vi "SP Adjust Limit with Waveform Data.vi"(7 "Limit":T1={"Parameter"={"Stimulus Port"=1, "Response Port"=1}, "Format"=enum."Log Mag", "Limit Type"=enum."Upper", "Points"=[], "Referential Limit"={"Ref Limit"=FALSE, "Ref Type"=enum."Current", "Model"="", "Serial"="", "Run Type"=enum."Most Recent", "Run"=0, "Field"="", "Field Value"=""}, "Limit #"=1} {"Parameter"."Stimulus Port" min=1 step=1; "Parameter"."Response Port" min=1 step=1}, 8 "error in (no error)":errorcluster, 9 "Data Waveform":waveform(dbl)={"t0"=timestamp(0 s since 1904-01-01), "dt"=0.0, "Y"=[]}, 10 "Frequency Waveform":waveform(dbl)={"t0"=timestamp(0 s since 1904-01-01), "dt"=0.0, "Y"=[]}) -> (0 "error out":errorcluster, 5 "Modified Limit":T1={"Parameter"={"Stimulus Port"=1, "Response Port"=1}, "Format"=enum."Log Mag", "Limit Type"=enum."Upper", "Points"=[], "Referential Limit"={"Ref Limit"=FALSE, "Ref Type"=enum."Current", "Model"="", "Serial"="", "Run Type"=enum."Most Recent", "Run"=0, "Field"="", "Field Value"=""}, "Limit #"=1} {"Parameter"."Stimulus Port" min=1 step=1; "Parameter"."Response Port" min=1 step=1})   [LabVIEW 2011]
uses:
  TypeDefs/SP Limit.ctl
  TypeDefs/SP Parameter.ctl
  TypeDefs/SP Format.ctl
  TypeDefs/SP Limit Type.ctl
  TypeDefs/SP Limit Point.ctl
  Test Referential Limit.ctl
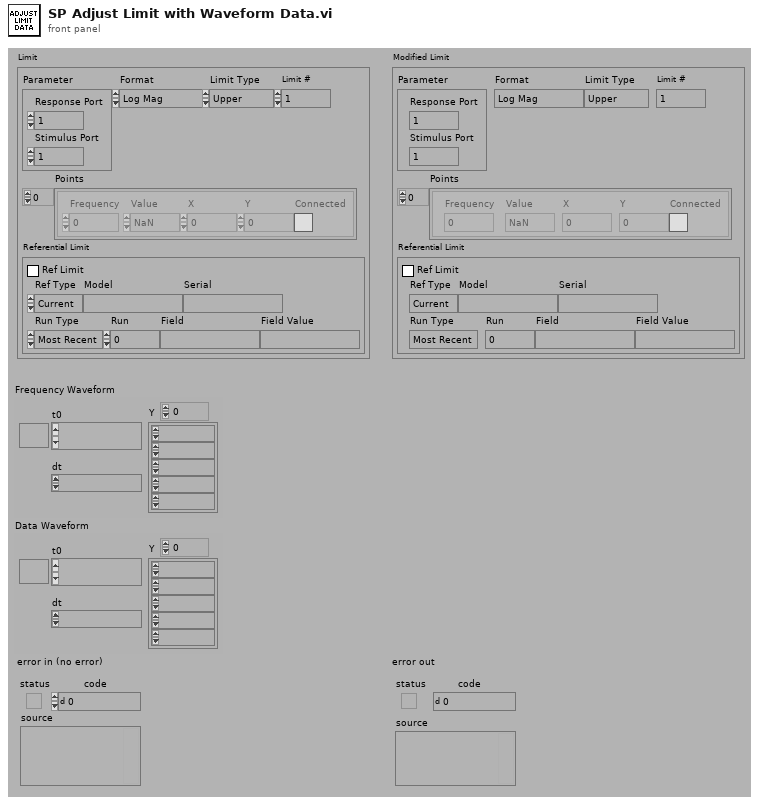
[diagram p1: front panel]
types:
  T1 = typedef "SP Limit.ctl" = cluster{"Parameter":T2, "Format":T3, "Limit Type":T4, "Points":T5[], "Referential Limit":T6, "Limit #":i8}
  T2 = typedef "SP Parameter.ctl" = cluster{"Stimulus Port":i8, "Response Port":i8}
  T3 = typedef "SP Format.ctl" = enum16{"Log Mag", "Lin Mag", "SWR", "Phase", "Expanded Phase", "Delay", "Insertion Loss", "Isolation", "Return Loss"}
  T4 = typedef "SP Limit Type.ctl" = enum16{"Upper", "Lower", "Delta", "Filter", "Referential"}
  T5 = typedef "SP Limit Point.ctl" = cluster{"Frequency":dbl, "Value":dbl, "X":dbl, "Y":dbl, "Connected":bool}
  T6 = typedef "Test Referential Limit.ctl" = cluster{"Ref Limit":bool, "Ref Type":enum16{"Current", "Specify"}, "Model":string, "Serial":string, "Run Type":enum16{"Most Recent", "Run #", "Match Field"}, "Run":i32, "Field":string, "Field Value":string}
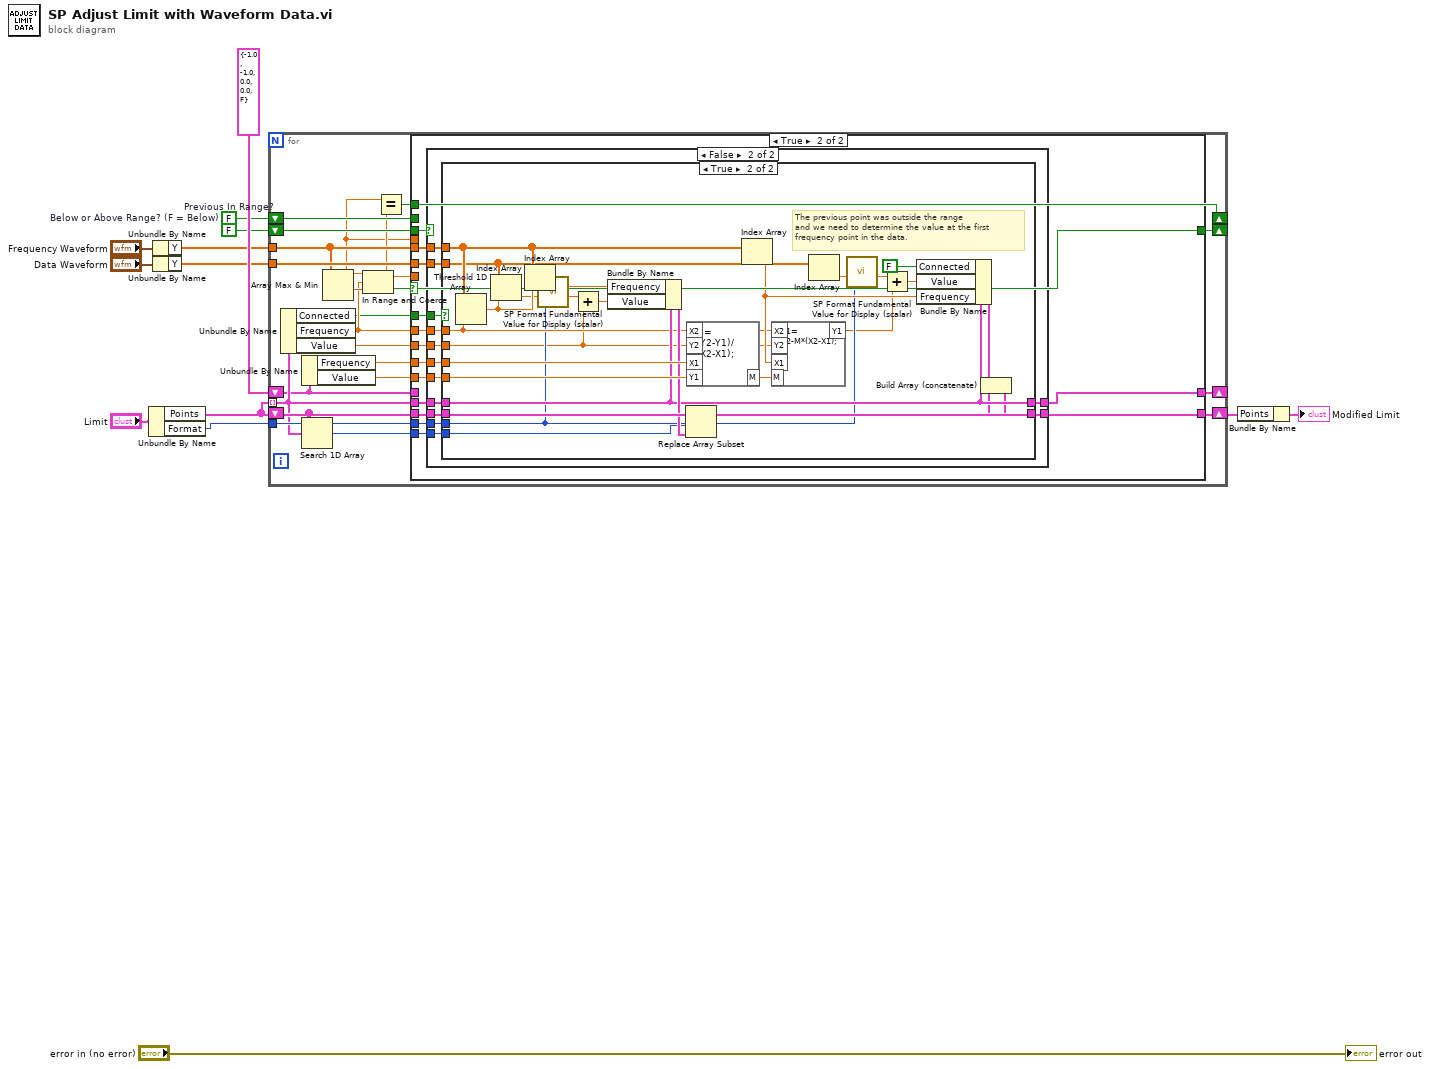
[diagram p0: block diagram]
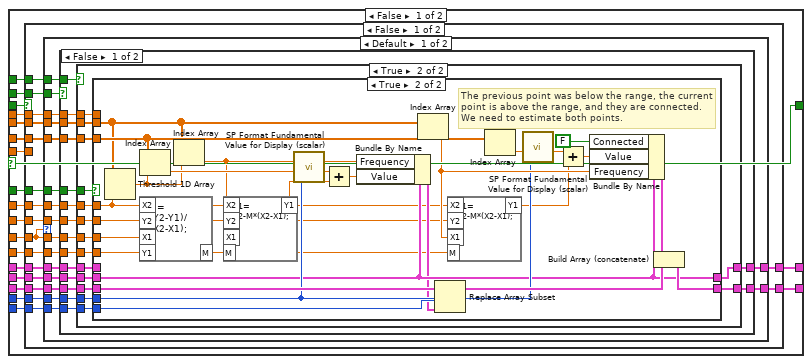
[diagram p2: hidden frame]
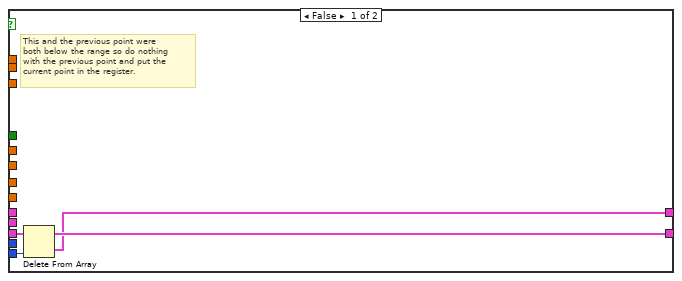
[diagram p3: hidden frame]
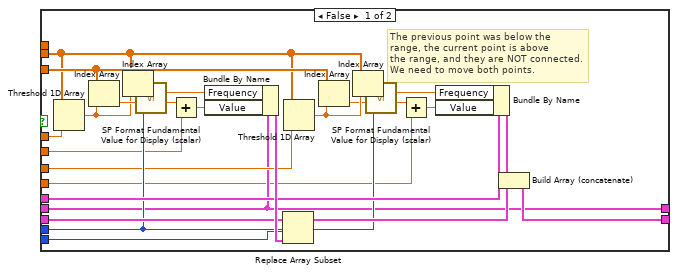
[diagram p4: hidden frame]
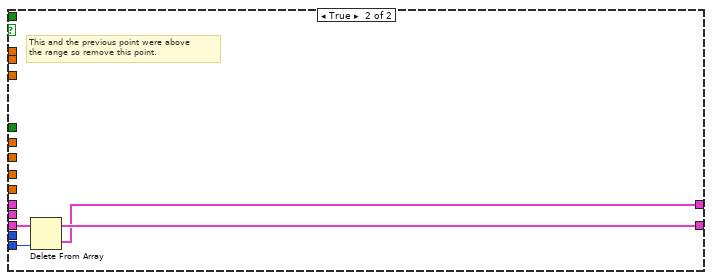
[diagram p5: hidden frame]
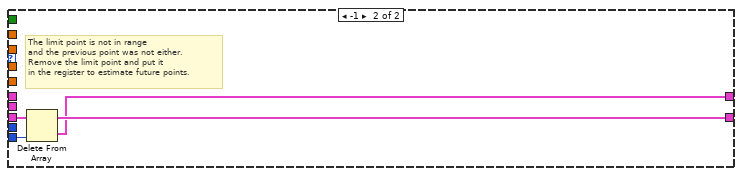
[diagram p6: hidden frame]
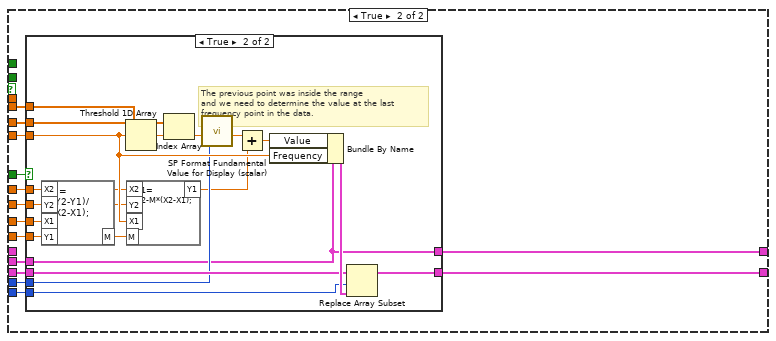
[diagram p7: hidden frame]
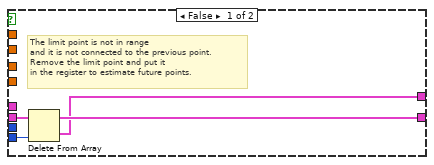
[diagram p8: hidden frame]
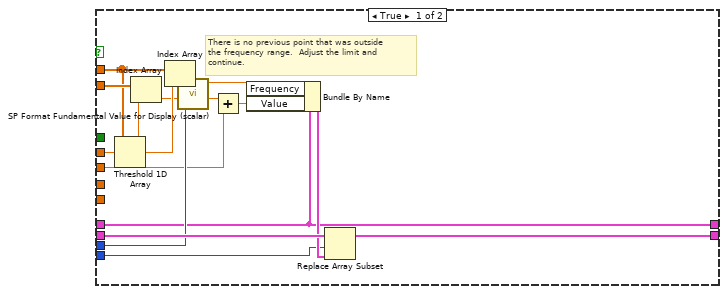
[diagram p9: hidden frame]
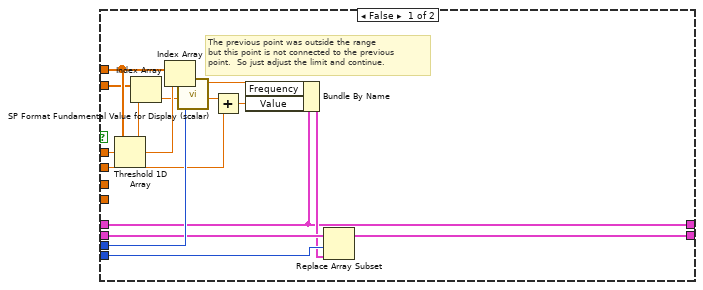
[diagram p10: hidden frame]
diagram:
  w2 = FALSE  # Below or Above Range? (F = Below)
  w3 = FALSE  # Previous In Range?
  n1 = Unbundle By Name("Limit") -> ("Points"=w7:T5[], "Format"=w6:T3)
  n2 = Unbundle By Name("Frequency Waveform") -> ("Y"=w4:dbl[])
  n3 = Unbundle By Name("Data Waveform") -> ("Y"=w1:dbl[])
  n4 = for {
    tunnel: w4 -> [w32]
    tunnel: w1 -> [w35]
    tunnel: w7 -> [w27] mode=indexing
    shift-right: [w33] -> w10
    shift-left: w7 -> [w26]
    tunnel: w6 -> [w28]
    shift-right: [w24] -> _
    shift-left: T5 {"Frequency"=-1.0, "Value"=-1.0, "X"=0.0, "Y"=0.0, "Connected"=FALSE} ("Point") -> [w14]
    shift-right: [w22] -> _
    shift-left: w3 -> [w23]
    shift-right: [w16] -> _
    shift-left: w2 -> [w18]
    n5 = Unbundle By Name(w27) -> ("Connected"=w19:bool, "Frequency"=w30:dbl, "Value"=w34:dbl)
    n6 = Unbundle By Name(w14) -> ("Frequency"=w21:dbl, "Value"=w20:dbl)
    n7 = Search 1D Array(1D array=w26, element=w27) -> (index of element=w25:i32)  [unwired: 1 out]
    n8 = Array Max & Min(array=w32) -> (max value=w15:dbl, min value=w31:dbl)  [unwired: 2 out]
    n9 = In Range and Coerce(upper limit=w15, x=w30, lower limit=w31) -> (coerced(x)=w17:dbl, In Range?=w29:bool)
    n10 = Equal?(x=w15, y=w17) -> (x = y?=w16:bool)
    n11 = case shown="True" w29 {
      selector: w29 -> [w41 w223]
      tunnel: w35 -> [w51 w236]
      tunnel: w34 -> [w54 w230]
      tunnel: w26 -> [w47 w232]
      tunnel: [w46 w231] -> w33
      tunnel: w32 -> [w50 w234]
      tunnel: w30 -> [w53 w235]
      tunnel: w27 -> [w55 w233]
      tunnel: w28 -> [w49 w229]
      tunnel: w25 -> [w48 w228]
      tunnel: [w45 w224] -> w24
      tunnel: w17 -> [w52 _]
      tunnel: w23 -> [w44 w227]
      tunnel: [w41 w223] -> w22
      tunnel: w21 -> [w42 w226]
      tunnel: w20 -> [w43 w225]
      tunnel: w19 -> [w40 w222]
      tunnel: w18 -> [w39 _]
      tunnel: w16 -> [w38 _]
      tunnel: w15 -> [w37 _]
      tunnel: w14 -> [w36 _]
      frame False {
        n12 = case shown="False" w44 {
          tunnel: w43 -> [w66 w188]
          tunnel: w55 -> [w58 w198]
          tunnel: w54 -> [w68 w197]
          tunnel: w53 -> [w67 w196]
          tunnel: w52 -> [_ w195]
          tunnel: w51 -> [w60 w194]
          tunnel: w50 -> [w59 w193]
          tunnel: w49 -> [w63 w192]
          tunnel: w48 -> [w69 w191]
          tunnel: w47 -> [w72 w190]
          tunnel: w42 -> [w65 w189]
          tunnel: [w71 w187] -> w46
          tunnel: [w70 w186] -> w45
          tunnel: w40 -> [w61 w185]
          tunnel: w39 -> [w64 _]
          tunnel: w38 -> [w62 _]
          tunnel: w37 -> [w57 _]
          tunnel: w36 -> [w56 _]
          frame False {
            n13 = case shown="Default" w65 {
              tunnel: w72 -> [w87 w184]
              tunnel: [w81 w183] -> w71
              tunnel: [w80 w182] -> w70
              tunnel: w69 -> [w89 w181]
              tunnel: w68 -> [w84 _]
              tunnel: w67 -> [w83 _]
              tunnel: w66 -> [w86 _]
              tunnel: w65 -> [w85 _]
              tunnel: w64 -> [w82 _]
              tunnel: w63 -> [w88 _]
              tunnel: w62 -> [w79 _]
              tunnel: w61 -> [w78 _]
              tunnel: w60 -> [w77 _]
              tunnel: w59 -> [w76 _]
              tunnel: w58 -> [w75 _]
              tunnel: w57 -> [w74 _]
              tunnel: w56 -> [w73 _]
              frame Default {
                n14 = case shown="False" w82 {
                  tunnel: w89 -> [w104 w179]
                  tunnel: w88 -> [w93 _]
                  tunnel: w87 -> [w105 w180]
                  tunnel: w86 -> [w96 _]
                  tunnel: w85 -> [w97 _]
                  tunnel: w84 -> [w98 _]
                  tunnel: w83 -> [w99 _]
                  tunnel: [w103 w178] -> w81
                  tunnel: [w102 w177] -> w80
                  tunnel: w79 -> [w101 _]
                  tunnel: w78 -> [w100 _]
                  tunnel: w77 -> [w95 _]
                  tunnel: w76 -> [w94 _]
                  tunnel: w75 -> [w92 _]
                  tunnel: w74 -> [w91 _]
                  tunnel: w73 -> [w90 _]
                  frame False {
                    n15 = case shown="True" w101 {
                      tunnel: w105 -> [w109 w122]
                      tunnel: w104 -> [w108 w124]
                      tunnel: [w107 w113] -> w103
                      tunnel: [w106 w110] -> w102
                      tunnel: w100 -> [_ w120]
                      tunnel: w99 -> [_ w116]
                      tunnel: w98 -> [_ w117]
                      tunnel: w97 -> [_ w118]
                      tunnel: w96 -> [_ w119]
                      tunnel: w95 -> [_ w114]
                      tunnel: w94 -> [_ w115]
                      tunnel: w93 -> [_ w123]
                      tunnel: w92 -> [_ w121]
                      tunnel: w91 -> [_ w112]
                      tunnel: w90 -> [_ w111]
                      frame False {
                        # "This and the previous point were\nboth below the range so do nothing\nwith the previous point and put the\ncurrent point in the register."
                        n16 = Delete From Array(array=w109, index=w108) -> (deleted portion=w106:T5, array with subset deleted=w107:T5[])  [unwired: 1 in]
                      }
                      frame True {
                        n17 = case shown="True" w120 {
                          tunnel: w124 -> [w143 w166]
                          tunnel: w123 -> [w133 w160]
                          tunnel: w122 -> [w144 w168]
                          tunnel: w121 -> [w129 w159]
                          tunnel: w119 -> [w125 w171]
                          tunnel: w118 -> [w130 w172]
                          tunnel: w117 -> [w127 w156]
                          tunnel: w116 -> [w142 w157]
                          tunnel: w115 -> [w131 w161]
                          tunnel: w114 -> [w132 w162]
                          tunnel: [w134 w169] -> w113
                          tunnel: w112 -> [_ _]
                          tunnel: w111 -> [w137 _]
                          tunnel: [w129 w159] -> w110
                          frame False {
                            # "The previous point was below the\nrange, the current point is above\nthe range, and they are NOT connected.\nWe need to move both points."
                            n18 = Threshold 1D Array(2:w142, 3:w131) -> (0:w146:dbl)  [unwired: 1 out]
                            n19 = Index Array(array=w132, index=w146) -> (element=w147:dbl)
                            n20 = Index Array(array=w131, index=w146) -> (element=w145:dbl)
                            n21 = call "SP Format Fundamental Value for Display (scalar).vi"("Format"=w133, "Stored Value (0, linear)"=w147) -> ("Display Value"=w148:dbl)  [unwired: 5 out]
                            n22 = Add(x=w148, y=w127) -> (x+y=w128:dbl)
                            n23 = Bundle By Name(cluster=w129, "Frequency"=w145, "Value"=w128) -> (w149:T5)
                            n24 = Replace Array Subset(array=w144, new element=w149, index=w143) -> (w135:T5[])
                            n25 = Threshold 1D Array(2:w130, 3:w131) -> (0:w140:dbl)  [unwired: 1 out]
                            n26 = Index Array(array=w132, index=w140) -> (element=w139:dbl)
                            n27 = Index Array(array=w131, index=w140) -> (element=w141:dbl)
                            n28 = call "SP Format Fundamental Value for Display (scalar).vi"("Format"=w133, "Stored Value (0, linear)"=w139) -> ("Display Value"=w138:dbl)  [unwired: 5 out]
                            n29 = Add(x=w138, y=w125) -> (x+y=w126:dbl)
                            n30 = Bundle By Name(cluster=w137, "Frequency"=w141, "Value"=w126) -> (w136:T5)
                            n31 = Build Array (concatenate)(w136, w135) -> (w134:T5[])
                          }
                          frame True {
                            # "The previous point was below the range, the current\npoint is above the range, and they are connected.\nWe need to estimate both points."
                            n32 = Threshold 1D Array(2:w157, 3:w161) -> (0:w163:dbl)  [unwired: 1 out]
                            n33 = Index Array(array=w162, index=w163) -> (element=w164:dbl)
                            n34 = formula code="M=\n(Y2-Y1)/(X2-X1);"("X2"=w157, "Y2"=w156, "X1"=w172, "Y1"=w171) -> ("M"=w155:dbl)
                            n35 = Index Array(array=w161, index=w163) -> (element=w154:dbl)
                            n36 = formula code="Y1=\nY2-M*(X2-X1);"("X2"=w157, "Y2"=w156, "X1"=w154, "M"=w155) -> ("Y1"=w152:dbl)
                            n37 = call "SP Format Fundamental Value for Display (scalar).vi"("Format"=w160, "Stored Value (0, linear)"=w164) -> ("Display Value"=w165:dbl)  [unwired: 5 out]
                            n38 = Add(x=w165, y=w152) -> (x+y=w153:dbl)
                            n39 = Bundle By Name(cluster=w159, "Frequency"=w154, "Value"=w153) -> (w158:T5)
                            n40 = Index Array(array=w161) -> (element=w175:dbl)  [unwired: 1 in]
                            n41 = Replace Array Subset(array=w168, new element=w158, index=w166) -> (w167:T5[])
                            n42 = formula code="Y1=\nY2-M*(X2-X1);"("X2"=w157, "Y2"=w156, "X1"=w175, "M"=w155) -> ("Y1"=w151:dbl)
                            n43 = Index Array(array=w162) -> (element=w174:dbl)  [unwired: 1 in]
                            n44 = call "SP Format Fundamental Value for Display (scalar).vi"("Format"=w160, "Stored Value (0, linear)"=w174) -> ("Display Value"=w173:dbl)  [unwired: 5 out]
                            n45 = Add(x=w173, y=w151) -> (x+y=w150:dbl)
                            n46 = Bundle By Name(cluster=w159, "Connected"=FALSE, "Value"=w150, "Frequency"=w175) -> (w170:T5)
                            n47 = Build Array (concatenate)(w170, w167) -> (w169:T5[])
                          }
                        }
                      }
                    }
                  }
                  frame True {
                    # "This and the previous point were above\nthe range so remove this point."
                    n48 = Delete From Array(array=w180, index=w179) -> (deleted portion=w177:T5, array with subset deleted=w178:T5[])  [unwired: 1 in]
                  }
                }
              }
              frame -1 {
                # "The limit point is not in range\nand the previous point was not either.\nRemove the limit point and put it\nin the register to estimate future points."
                n49 = Delete From Array(array=w184, index=w181) -> (deleted portion=w182:T5, array with subset deleted=w183:T5[])  [unwired: 1 in]
              }
            }
          }
          frame True {
            n50 = case shown="True" w185 {
              tunnel: w194 -> [_ w213]
              tunnel: w196 -> [_ w211]
              tunnel: w193 -> [_ w214]
              tunnel: w198 -> [_ w205]
              tunnel: w190 -> [w202 w215]
              tunnel: [w201 w216] -> w187
              tunnel: w197 -> [_ w210]
              tunnel: w192 -> [_ w208]
              tunnel: w191 -> [w199 w209]
              tunnel: w189 -> [_ w207]
              tunnel: w195 -> [_ w212]
              tunnel: w188 -> [_ w206]
              tunnel: [w200 w205] -> w186
              frame False {
                # "The limit point is not in range\nand it is not connected to the previous point.\nRemove the limit point and put it\nin the register to estimate future points."
                n51 = Delete From Array(array=w202, index=w199) -> (deleted portion=w200:T5, array with subset deleted=w201:T5[])  [unwired: 1 in]
              }
              frame True {
                # "The previous point was inside the range\nand we need to determine the value at the last\nfrequency point in the data."
                n52 = formula code="M=\n(Y2-Y1)/(X2-X1);"("X2"=w211, "Y2"=w210, "X1"=w207, "Y1"=w206) -> ("M"=w217:dbl)
                n53 = Threshold 1D Array(2:w212, 3:w214) -> (0:w218:dbl)  [unwired: 1 out]
                n54 = formula code="Y1=\nY2-M*(X2-X1);"("X2"=w211, "Y2"=w210, "X1"=w212, "M"=w217) -> ("Y1"=w203:dbl)
                n55 = Index Array(array=w213, index=w218) -> (element=w220:dbl)
                n56 = call "SP Format Fundamental Value for Display (scalar).vi"("Format"=w208, "Stored Value (0, linear)"=w220) -> ("Display Value"=w219:dbl)  [unwired: 5 out]
                n57 = Add(x=w219, y=w203) -> (x+y=w204:dbl)
                n58 = Bundle By Name(cluster=w205, "Value"=w204, "Frequency"=w212) -> (w221:T5)
                n59 = Replace Array Subset(array=w215, new element=w221, index=w209) -> (w216:T5[])
              }
            }
          }
        }
      }
      frame True {
        n60 = case shown="False" w227 {
          tunnel: w236 -> [w251 w260]
          tunnel: w235 -> [w250 w263]
          tunnel: w234 -> [w249 w255]
          tunnel: w233 -> [w239 w254]
          tunnel: w232 -> [w247 w258]
          tunnel: [w246 w257] -> w231
          tunnel: w230 -> [w238 w262]
          tunnel: w229 -> [w241 w259]
          tunnel: w228 -> [w240 w256]
          tunnel: w226 -> [_ w261]
          tunnel: w225 -> [_ w264]
          tunnel: [w239 w252] -> w224
          tunnel: w222 -> [_ w253]
          frame True {
            # "There is no previous point that was outside\nthe frequency range.  Adjust the limit and\ncontinue."
            n61 = Threshold 1D Array(2:w250, 3:w249) -> (0:w244:dbl)  [unwired: 1 out]
            n62 = Index Array(array=w251, index=w244) -> (element=w243:dbl)
            n63 = Index Array(array=w249, index=w244) -> (element=w248:dbl)
            n64 = call "SP Format Fundamental Value for Display (scalar).vi"("Format"=w241, "Stored Value (0, linear)"=w243) -> ("Display Value"=w242:dbl)  [unwired: 5 out]
            n65 = Add(x=w242, y=w238) -> (x+y=w237:dbl)
            n66 = Bundle By Name(cluster=w239, "Frequency"=w248, "Value"=w237) -> (w245:T5)
            n67 = Replace Array Subset(array=w247, new element=w245, index=w240) -> (w246:T5[])
          }
          frame False {
            n68 = case shown="True" w253 {
              tunnel: w264 -> [_ w305]
              tunnel: w263 -> [w270 w290]
              tunnel: w262 -> [w266 w283]
              tunnel: w261 -> [_ w303]
              tunnel: w260 -> [w271 w289]
              tunnel: w259 -> [w274 w288]
              tunnel: w258 -> [w273 w293]
              tunnel: [w267 w285] -> w257
              tunnel: w256 -> [w275 w287]
              tunnel: w255 -> [w272 w291]
              tunnel: w254 -> [w268 w292]
              tunnel: [w268 w292] -> w252
              frame False {
                # "The previous point was outside the range\nbut this point is not connected to the previous\npoint.  So just adjust the limit and continue."
                n69 = Threshold 1D Array(2:w270, 3:w272) -> (0:w278:dbl)  [unwired: 1 out]
                n70 = Index Array(array=w271, index=w278) -> (element=w277:dbl)
                n71 = Index Array(array=w272, index=w278) -> (element=w279:dbl)
                n72 = call "SP Format Fundamental Value for Display (scalar).vi"("Format"=w274, "Stored Value (0, linear)"=w277) -> ("Display Value"=w276:dbl)  [unwired: 5 out]
                n73 = Add(x=w276, y=w266) -> (x+y=w265:dbl)
                n74 = Bundle By Name(cluster=w268, "Frequency"=w279, "Value"=w265) -> (w269:T5)
                n75 = Replace Array Subset(array=w273, new element=w269, index=w275) -> (w267:T5[])
              }
              frame True {
                # "The previous point was outside the range\nand we need to determine the value at the first\nfrequency point in the data."
                n76 = Threshold 1D Array(2:w290, 3:w291) -> (0:w297:dbl)  [unwired: 1 out]
                n77 = Index Array(array=w289, index=w297) -> (element=w296:dbl)
                n78 = Index Array(array=w291, index=w297) -> (element=w298:dbl)
                n79 = call "SP Format Fundamental Value for Display (scalar).vi"("Format"=w288, "Stored Value (0, linear)"=w296) -> ("Display Value"=w295:dbl)  [unwired: 5 out]
                n80 = Add(x=w295, y=w283) -> (x+y=w282:dbl)
                n81 = Bundle By Name(cluster=w292, "Frequency"=w298, "Value"=w282) -> (w294:T5)
                n82 = Replace Array Subset(array=w293, new element=w294, index=w287) -> (w286:T5[])
                n83 = formula code="M=\n(Y2-Y1)/(X2-X1);"("X2"=w290, "Y2"=w283, "X1"=w303, "Y1"=w305) -> ("M"=w304:dbl)
                n84 = Index Array(array=w291) -> (element=w300:dbl)  [unwired: 1 in]
                n85 = formula code="Y1=\nY2-M*(X2-X1);"("X2"=w290, "Y2"=w283, "X1"=w300, "M"=w304) -> ("Y1"=w281:dbl)
                n86 = Index Array(array=w289) -> (element=w301:dbl)  [unwired: 1 in]
                n87 = call "SP Format Fundamental Value for Display (scalar).vi"("Format"=w288, "Stored Value (0, linear)"=w301) -> ("Display Value"=w302:dbl)  [unwired: 5 out]
                n88 = Add(x=w302, y=w281) -> (x+y=w280:dbl)
                n89 = Bundle By Name(cluster=w292, "Connected"=FALSE, "Value"=w280, "Frequency"=w300) -> (w284:T5)
                n90 = Build Array (concatenate)(w284, w286) -> (w285:T5[])
              }
            }
          }
        }
      }
    }
  }
  n91 = Bundle By Name(cluster="Limit", "Points"=w10) -> (→"Modified Limit":T1)
  "error out" <- "error in (no error)"
